vi "docmd1.vi"(4 "Elements":string[](array[string]), 5 "lowercase file ext":string, 6 "DevNo":i32, 7 "CMDpath":path) -> (0 "rezult":string, 2 "time stamp":timestamp, 3 "date_time":string)   [LabVIEW 2010]
uses:
  <vilib>/Utility/miscctls.llb/LVDateTimeRec.ctl
  <vilib>/Utility/error.llb/DialogType.ctl
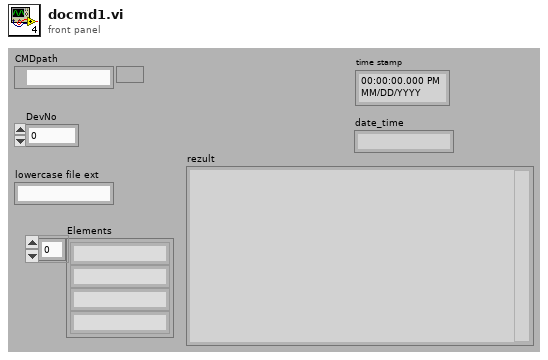
[diagram p1: front panel]
types:
  T1 = cluster{"DevNo":i32, "Cmd":string, "Param":string}
  T2 = typedef "LVDateTimeRec.ctl" = cluster{"fractional second":dbl, "second":i32, "minute":i32, "hour":i32, "day of month":i32, "month":i32, "year":i32, "day of week":i32, "day of year":i32, "DST":i32}
  T3 = typedef "DialogType.ctl" = u16
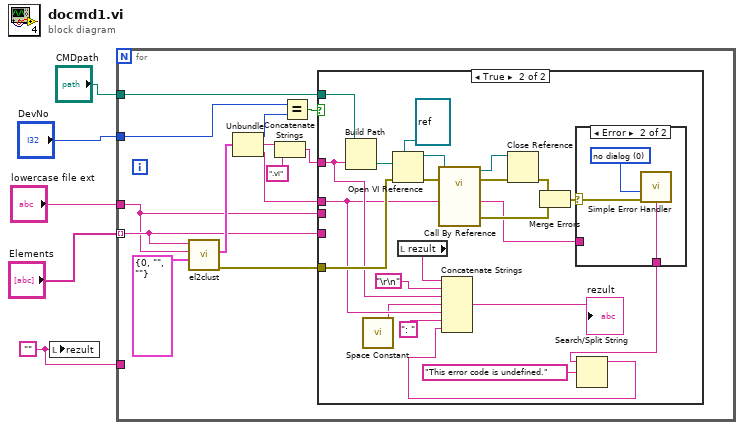
[diagram p0: block diagram]
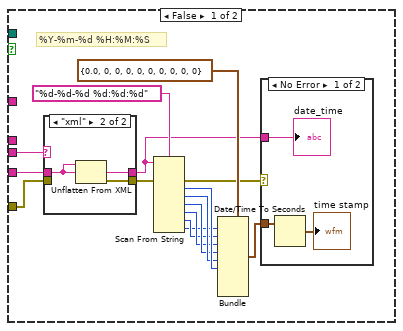
[diagram p2: hidden frame]
diagram:
  w1 = ""
  n1 = local write "rezult"(w1) -> ()
  n2 = for {
    tunnel: "Elements" -> [w11] mode=indexing
    tunnel: "lowercase file ext" -> [w10]
    tunnel: "DevNo" -> [w7]
    tunnel: "CMDpath" -> [w6]
    tunnel: w1 -> [_]
    n3 = call "el2clust.vi"("Cluster in"=T1 {"DevNo"=0, "Cmd"="", "Param"=""}, "type"=w10, "element"=w11) -> ("error out 2"=w16:errorcluster, "Cluster"=w17:T1)  [unwired: 3 in]
    n4 = Unbundle(w17) -> ("DevNo"=w18:i32, "Cmd"=w14:string, "Param"=w13:string)
    n5 = Concatenate Strings(w14, ".vi" ("string")) -> (w12:string)
    n6 = Equal?(x=w7, y=w18) -> (x = y?=w15:bool)
    n7 = case shown="True" w15 {
      tunnel: w13 -> [_ w52]
      tunnel: w16 -> [w19 w63]
      tunnel: w12 -> [_ w54]
      tunnel: w11 -> [w33 _]
      tunnel: w10 -> [w32 _]
      tunnel: w6 -> [_ w53]
      frame False {
        # "%Y-%m-%d %H:%M:%S"
        n8 = case shown="\"xml\"" w32 {
          tunnel: w19 -> [w38 _]
          tunnel: w33 -> [w37 w41]
          tunnel: [w37 w40] -> w21
          tunnel: [w38 w39] -> w20
          frame "txt", Default {
          }
          frame "xml" {
            n9 = Unflatten From XML(xml string=w41, type=w41) -> (value=w40:string, error out=w39:errorcluster)  [unwired: 1 in]
          }
        }
        n10 = Scan From String(format string="%d-%d-%d %d:%d:%d" ("time format string (%c)"), input string=w21, error in=w20) -> (error out=w22:errorcluster, output 1=w30:i32, output 2=w29:i32, output 3=w28:i32, output 4=w27:i32, output 5=w26:i32, output 6=w25:i32)  [unwired: 7 in, 2 out]
        n11 = Bundle(cluster=T2 {"fractional second"=0.0, "second"=0, "minute"=0, "hour"=0, "day of month"=0, "month"=0, "year"=0, "day of week"=0, "day of year"=0, "DST"=0} ("date time rec"), "second"=w25, "minute"=w26, "hour"=w27, "day of month"=w28, "month"=w29, "year"=w30) -> (w23:T2)  [unwired: 4 in]
        n12 = case shown="No Error" w22 {
          tunnel: w23 -> [w36 _]
          tunnel: w21 -> [w35 _]
          frame No Error {
            n13 = Date/Time To Seconds(2:w36) -> (0:→"time stamp":timestamp)  [unwired: 1 in]
            "date_time" <- w35
          }
          frame Error {
          }
        }
      }
      frame True {
        n14 = Build Path(base path=w53, name or relative path=w54) -> (appended path=w56:path)
        n15 = call <vilib>:"Space Constant.vi"() -> ("String"=w51:string)
        n16 = Open VI Reference(type specifier VI Refnum (for type only)=refnum<vi> refnum, vi path=w56, error in (no error)=w63) -> (vi reference=w61:refnum<vi>, error out=w60:errorcluster)  [unwired: 3 in]
        n17 = local read "rezult"() -> (w46:string)
        n18 = call-by-ref "?"(reference=w61, error in=w60, "Param"=w52) -> (reference out=w62:refnum<vi>, error out=w59:errorcluster, 0:"error out"=w57:errorcluster, "Rezult"=w48:string)  [unwired: 5 in]
        n19 = Close Reference(reference=w62, error in (no error)=w59) -> (error out=w58:errorcluster)
        n20 = Merge Errors(w58, w57) -> (w49:errorcluster)
        n21 = case shown="Error" w49 {
          selector: w49 -> [_ w67]
          tunnel: [w64 w66] -> w44
          tunnel: w48 -> [w64 _]
          frame No Error {
          }
          frame Error {
            w65 = T3 0 items=["no dialog", "OK message", "continue or stop message", "OK message + warnings", "continue/stop + warnings"] ("type of dialog (OK msg:1)")
            n22 = call <vilib>:"Simple Error Handler.vi"("type of dialog (OK msg:1)"=w65, "error in (no error)"=w67) -> ("message"=w66:string)  [unwired: 3 in, 4 out]
          }
        }
        n23 = Search/Split String(string=w44, search string/char (-)="This error code is undefined.") -> (substring before match=w42:string)  [unwired: 1 in, 2 out]
        n24 = Concatenate Strings(w46, "\r\n", w54, w51, w52, ": " ("string"), w42) -> (→"rezult":string)
      }
    }
  }
